vi "FirstLastAvg.vi"(1 "waveform":waveform(dbl)={"t0"=timestamp(3462274995.8440003 s since 1904-01-01), "dt"=1.428e-05, "Y"=array[8000 elements]}) -> (0 "avg value":dbl=2.999278448848586)   [LabVIEW 2010]
uses:
  <vilib>/Analysis/NI_AALBase.lvlib
panel:
  out "Last Point Amplitude":dbl=2.9605986361275427
  out "First Point Amplitude":dbl=3.0374657435459085
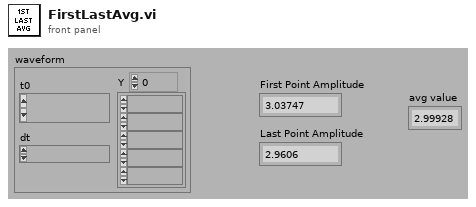
[diagram p1: front panel]
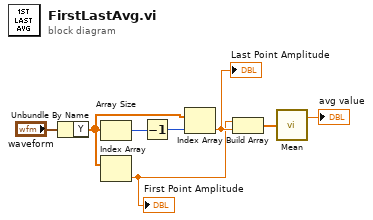
[diagram p0: block diagram]
diagram:
  n1 = Unbundle By Name("waveform") -> ("Y"=w5:dbl[])
  n2 = Array Size(array=w5) -> (size(s)=w3:i32)
  n3 = Index Array(array=w5) -> (element=w6:dbl)  [unwired: 1 in]
  "First Point Amplitude" <- w6
  n4 = Decrement(x=w3) -> (x-1=w4:i32)
  n5 = Index Array(array=w5, index=w4) -> (element=w7:dbl)
  "Last Point Amplitude" <- w7
  n6 = Build Array(w6, w7) -> (w2:dbl[])
  n7 = call <vilib>:"Mean.vi"("X"=w2) -> ("mean"=→"avg value":dbl)  [unwired: 1 out]
